vi "Read Displayed Data.vi"(8 "error in (no error)":errorcluster, 11 "VISA resource name":refnum<visa-resource-name>) -> (0 "error out":errorcluster, 2 "Displayed Data":T1, 3 "VISA resource name out":refnum<visa-resource-name>)   [LabVIEW 2015, in "Fluke 289.lvlib"]
doc: "Reads the present data that is displayed on the LCD display (not including the bargraph)."
uses:
  <instrlib>/Fluke 289/Fluke 289.lvlib
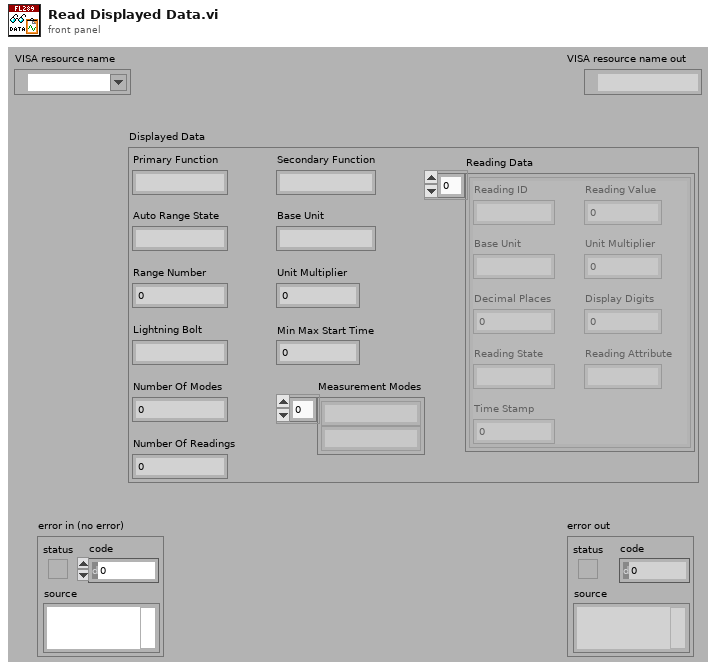
[diagram p1: front panel]
types:
  T1 = cluster{"Primary Function":string, "Secondary Function":string, "Auto Range State":string, "Base Unit":string, "Range Number":i32, "Unit Multiplier":i32, "Lightning Bolt":string, "Min Max Start Time":dbl, "Number Of Modes":i32, "Number Of Readings":i32, "Measurement Modes":string[], "Reading Data":cluster{"Reading ID":string, "Reading Value":dbl, "Base Unit":string, "Unit Multiplier":i32, "Decimal Places":i32, "Display Digits":i32, "Reading State":string, "Reading Attribute":string, "Time Stamp":dbl}[]}
  T2 = cluster{"Reading ID":string, "Reading Value":dbl, "Base Unit":string, "Unit Multiplier":i32, "Decimal Places":i32, "Display Digits":i32, "Reading State":string, "Reading Attribute":string, "Time Stamp":dbl}
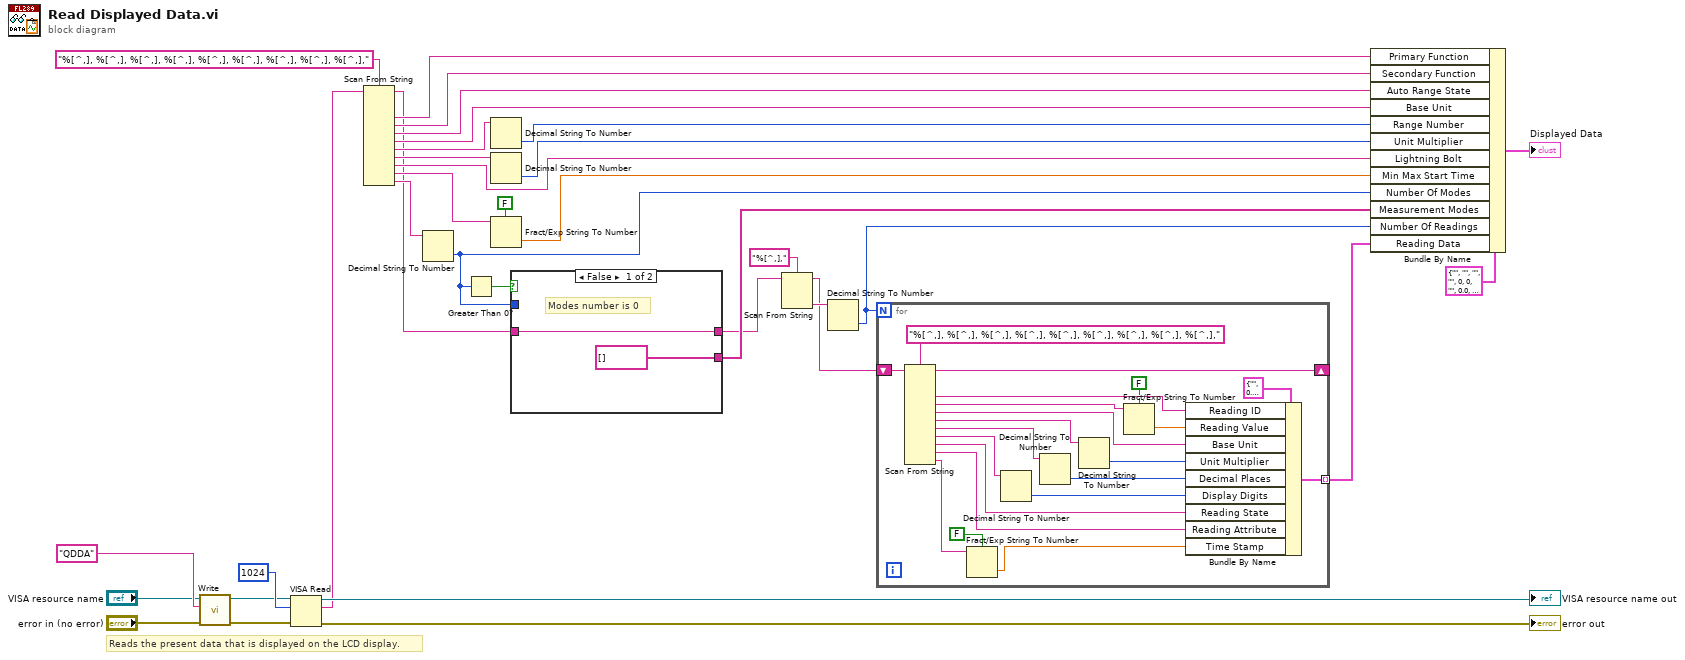
[diagram p0: block diagram]
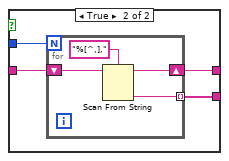
[diagram p2: hidden frame]
diagram:
  # "Reads the present data that is displayed on the LCD display."
  n1 = call <instrlib>:"Write.vi"("error in (no error)"="error in (no error)", "Write Buffer"="QDDA", "VISA resource name"="VISA resource name") -> ("error out"=w30:errorcluster, "VISA resource name out"=w31:refnum<visa-resource-name>)  [unwired: 7 in]
  n2 = VISA Read(VISA resource name=w31, byte count=u32 1024, error in (no error)=w30) -> (VISA resource name out=→"VISA resource name out":refnum<visa-resource-name>, read buffer=w26:string, error out=→"error out":errorcluster)  [unwired: 1 out]
  n3 = Scan From String(format string="%[^,], %[^,], %[^,], %[^,], %[^,], %[^,], %[^,], %[^,], %[^,],", input string=w26) -> (remaining string=w11:string, output 1=w25:string, output 2=w24:string, output 3=w23:string, output 4=w22:string, output 5=w21:string, output 6=w19:string, output 7=w16:string, output 8=w15:string, output 9=w13:string)  [unwired: 11 in, 2 out]
  n4 = Decimal String To Number(string=w13) -> (number=w9:i32)  [unwired: 2 in, 1 out]
  n5 = Greater Than 0?(x=w9) -> (x > 0?=w10:bool)
  n6 = Decimal String To Number(string=w21) -> (number=w20:i32)  [unwired: 2 in, 1 out]
  n7 = Decimal String To Number(string=w19) -> (number=w18:i32)  [unwired: 2 in, 1 out]
  n8 = Fract/Exp String To Number(use system decimal point (T)=FALSE, string=w15) -> (number=w17:dbl)  [unwired: 2 in, 1 out]
  n9 = case shown="False" w10 {
    tunnel: w11 -> [w37 w40]
    tunnel: [w37 w39] -> w6
    tunnel: w9 -> [_ w41]
    tunnel: [string[] [] w38] -> w8
    frame False {
      # "Modes number is 0"
    }
    frame True {
      n10 = for {
        N: w41 -> [_]
        shift-right: [w44] -> w39
        shift-left: w40 -> [w45]
        tunnel: [w42] -> w38 mode=indexing
        n11 = Scan From String(format string="%[^,],", input string=w45) -> (remaining string=w44:string, output 1=w42:string)  [unwired: 3 in, 2 out]
      }
    }
  }
  n12 = Scan From String(format string="%[^,],", input string=w6) -> (remaining string=w2:string, output 1=w5:string)  [unwired: 3 in, 2 out]
  n13 = Decimal String To Number(string=w5) -> (number=w4:i32)  [unwired: 2 in, 1 out]
  n14 = for {
    N: w4 -> [_]
    shift-right: [w65] -> _
    shift-left: w2 -> [w66]
    tunnel: [w63] -> w3 mode=indexing
    n15 = Scan From String(format string="%[^,], %[^,], %[^,], %[^,], %[^,], %[^,], %[^,], %[^,], %[^,],", input string=w66) -> (remaining string=w65:string, output 1=w61:string, output 2=w59:string, output 3=w58:string, output 4=w56:string, output 5=w54:string, output 6=w52:string, output 7=w51:string, output 8=w50:string, output 9=w49:string)  [unwired: 11 in, 2 out]
    n16 = Fract/Exp String To Number(use system decimal point (T)=FALSE, string=w49) -> (number=w47:dbl)  [unwired: 2 in, 1 out]
    n17 = Decimal String To Number(string=w52) -> (number=w53:i32)  [unwired: 2 in, 1 out]
    n18 = Decimal String To Number(string=w54) -> (number=w55:i32)  [unwired: 2 in, 1 out]
    n19 = Decimal String To Number(string=w56) -> (number=w57:i32)  [unwired: 2 in, 1 out]
    n20 = Fract/Exp String To Number(use system decimal point (T)=FALSE, string=w59) -> (number=w60:dbl)  [unwired: 2 in, 1 out]
    n21 = Bundle By Name(cluster=T2 {"Reading ID"="", "Reading Value"=0.0, "Base Unit"="", "Unit Multiplier"=0, "Decimal Places"=0, "Display Digits"=0, "Reading State"="", "Reading Attribute"="", "Time Stamp"=0.0} ("Reading Data"), "Reading ID"=w61, "Reading Value"=w60, "Base Unit"=w58, "Unit Multiplier"=w57, "Decimal Places"=w55, "Display Digits"=w53, "Reading State"=w51, "Reading Attribute"=w50, "Time Stamp"=w47) -> (w63:T2)
  }
  n22 = Bundle By Name(cluster=T1 {"Primary Function"="", "Secondary Function"="", "Auto Range State"="", "Base Unit"="", "Range Number"=0, "Unit Multiplier"=0, "Lightning Bolt"="", "Min Max Start Time"=0.0, "Number Of Modes"=0, "Number Of Readings"=0, "Measurement Modes"=[], "Reading Data"=[]} ("output cluster"), "Primary Function"=w25, "Secondary Function"=w24, "Auto Range State"=w23, "Base Unit"=w22, "Range Number"=w20, "Unit Multiplier"=w18, "Lightning Bolt"=w16, "Min Max Start Time"=w17, "Number Of Modes"=w9, "Measurement Modes"=w8, "Number Of Readings"=w4, "Reading Data"=w3) -> (→"Displayed Data":T1)
